vi "txt_to_int.vi"() -> ()   [LabVIEW 2019]
panel:
  out "white score":i32
  out "yellow score":i32
  out "red score":i32
  out "Cluster":T1
  in  "pos.txt":string
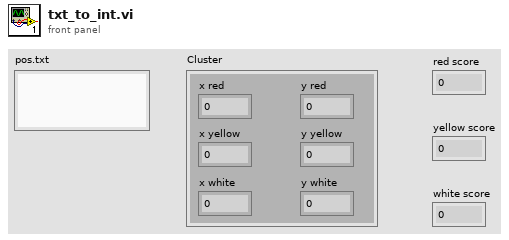
[diagram p1: front panel]
types:
  T1 = cluster{"x red":i32, "y red":i32, "x yellow":i32, "y yellow":i32, "x white":i32, "y white":i32}
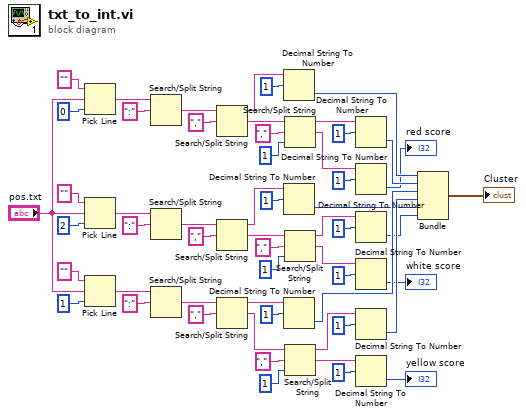
[diagram p0: block diagram]
diagram:
  n1 = Pick Line(string ("")="", multi-line string="pos.txt", line index=0) -> (output string=w49:string)
  n2 = Pick Line(string ("")="", multi-line string="pos.txt", line index=2) -> (output string=w11:string)
  n3 = Pick Line(string ("")="", multi-line string="pos.txt", line index=1) -> (output string=w12:string)
  n4 = Search/Split String(string=w49, search string/char (-)=":") -> (match + rest of string=w45:string)  [unwired: 1 in, 2 out]
  n5 = Search/Split String(string=w11, search string/char (-)=":") -> (match + rest of string=w21:string)  [unwired: 1 in, 2 out]
  n6 = Search/Split String(string=w12, search string/char (-)=":") -> (match + rest of string=w33:string)  [unwired: 1 in, 2 out]
  n7 = Search/Split String(string=w45, search string/char (-)=",") -> (substring before match=w44:string, match + rest of string=w43:string)  [unwired: 1 in, 1 out]
  n8 = Search/Split String(string=w21, search string/char (-)=",") -> (substring before match=w20:string, match + rest of string=w19:string)  [unwired: 1 in, 1 out]
  n9 = Search/Split String(string=w33, search string/char (-)=",") -> (substring before match=w32:string, match + rest of string=w31:string)  [unwired: 1 in, 1 out]
  n10 = Decimal String To Number(string=w44, offset=1) -> (number=w10:i32)  [unwired: 1 in, 1 out]
  n11 = Decimal String To Number(string=w20, offset=1) -> (number=w6:i32)  [unwired: 1 in, 1 out]
  n12 = Decimal String To Number(string=w32, offset=1) -> (number=w8:i32)  [unwired: 1 in, 1 out]
  n13 = Search/Split String(string=w43, search string/char (-)=",", offset (0)=1) -> (substring before match=w40:string, match + rest of string=w38:string)  [unwired: 1 out]
  n14 = Search/Split String(string=w19, search string/char (-)=",", offset (0)=1) -> (substring before match=w16:string, match + rest of string=w14:string)  [unwired: 1 out]
  n15 = Search/Split String(string=w31, search string/char (-)=",", offset (0)=1) -> (substring before match=w28:string, match + rest of string=w26:string)  [unwired: 1 out]
  n16 = Decimal String To Number(string=w40, offset=1) -> (number=w9:i32)  [unwired: 1 in, 1 out]
  n17 = Decimal String To Number(string=w38, offset=1) -> (number=→"red score":i32)  [unwired: 1 in, 1 out]
  n18 = Decimal String To Number(string=w16, offset=1) -> (number=w5:i32)  [unwired: 1 in, 1 out]
  n19 = Decimal String To Number(string=w14, offset=1) -> (number=→"white score":i32)  [unwired: 1 in, 1 out]
  n20 = Decimal String To Number(string=w28, offset=1) -> (number=w7:i32)  [unwired: 1 in, 1 out]
  n21 = Decimal String To Number(string=w26, offset=1) -> (number=→"yellow score":i32)  [unwired: 1 in, 1 out]
  n22 = Bundle(w10, w9, w8, w7, w6, w5) -> (→"Cluster":cluster{i32, i32, i32, i32, i32, i32})  [unwired: 1 in]
